vi "Turbo_encoder.vi"(8 "error in":errorcluster, 10 "input":dbl[](array[numeric]), 11 "Path In":path) -> (0 "error out":errorcluster, 2 "coded_data":dbl[](array[numeric]), 3 "Path Out":path)   [LabVIEW 2015]
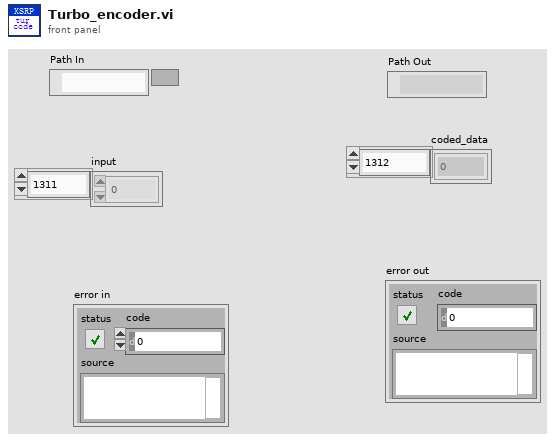
[diagram p1: front panel]
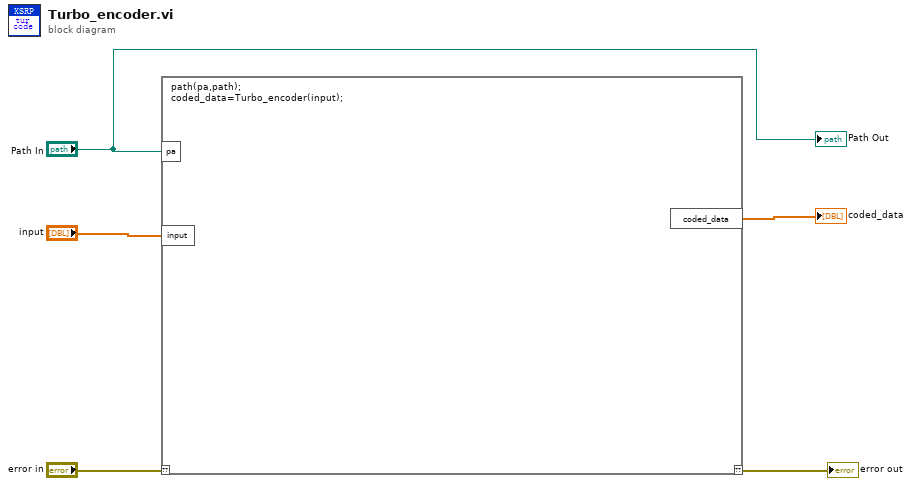
[diagram p0: block diagram]
diagram:
  n1 = script code="path(pa,path);\ncoded_data=Turbo_encoder(input);"("??"="error in", "pa"="Path In", "input"="input") -> ("??"=→"error out":errorcluster, "coded_data"=→"coded_data":dbl[])
  "Path Out" <- "Path In"
